vi "response to error.vi"(8 "error in":errorcluster, 11 "message from engine":T1) -> (0 "error out":errorcluster)   [LabVIEW 2013, in "Standard Engine Runtime.lvclass"]
uses:
  Standard Engine Runtime.lvclass
  main engine/message from engine.ctl
  main engine/message response type.ctl
  main engine/main engine.lvlib
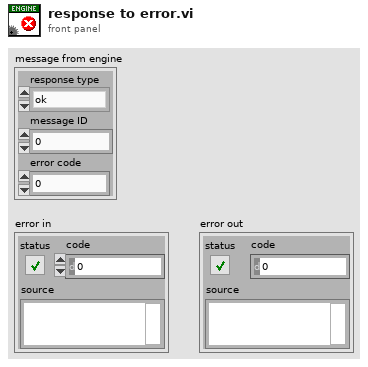
[diagram p1: front panel]
types:
  T1 = typedef "main engine.lvlib/message from engine.ctl" = cluster{"response type":T2, "message ID":u8, "error code":i32}
  T2 = typedef "main engine.lvlib/message response type.ctl" = enum8{"ok", "error"}
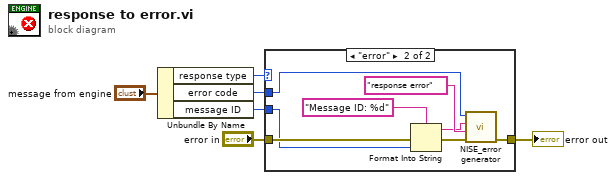
[diagram p0: block diagram]
diagram:
  n1 = Unbundle By Name("message from engine") -> ("response type"=w5:T2, "error code"=w1:i32, "message ID"=w2:u8)
  n2 = case shown="\"error\"" w5 {
    tunnel: "error in" -> [w7 w15]
    tunnel: [w7 w14] -> w3
    tunnel: w2 -> [_ w11]
    tunnel: w1 -> [_ w8]
    frame "ok" {
    }
    frame "error" {
      n3 = Format Into String(format string="Message ID: %d", error in=w15, w11) -> (resulting string=w10:string, error out=w12:errorcluster)  [unwired: 1 in]
      n4 = call <vilib>:"NISE_error generator.vi"("error in"=w12, "source"="response error", "append error message"=w10, "error code (0)"=w8) -> ("error out"=w14:errorcluster)  [unwired: 5 in]
    }
  }
  "error out" <- w3
